vi "Print Position.vi"(11 "positions":dbl[](array[numeric])) -> (3 "String":string)   [LabVIEW 2020, in "Manipulator.lvlib"]
uses:
  Manipulator.lvlib
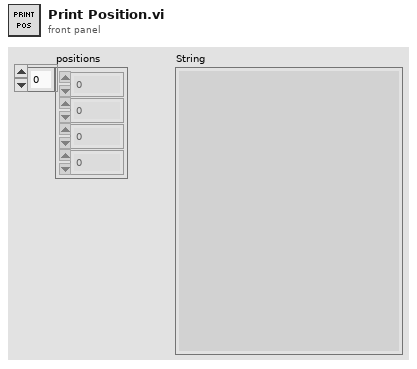
[diagram p1: front panel]
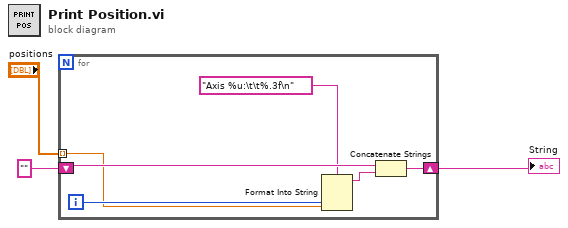
[diagram p0: block diagram]
diagram:
  n1 = for {
    tunnel: "positions" -> [w4] mode=indexing
    shift-right: [w8] -> w3
    shift-left: "" -> [w9]
    i -> [w5]
    n2 = Format Into String(format string="Axis %u:\t\t%.3f\n", w5, w4) -> (resulting string=w7:string)  [unwired: 2 in, 1 out]
    n3 = Concatenate Strings(w9, w7) -> (w8:string)
  }
  "String" <- w3
